vi "SRV_Strip Error if Matching Code.vi"(3 "error in (no error)":errorcluster, 4 "Strip Codes":i32[](array[numeric])) -> (10 "error out":errorcluster)   [LabVIEW 2014]
doc: "Strips the error if \"error in (code)\" matches one of the Strip Codes.\n\n\nAuthor: Mike Schultz - Logic PD"
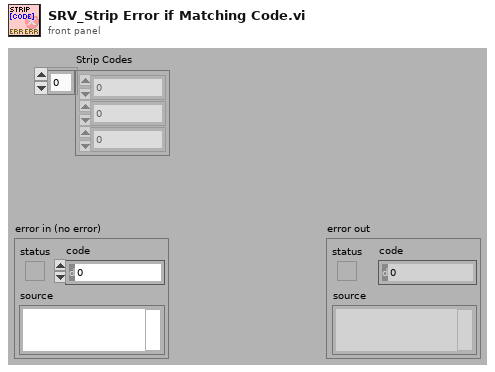
[diagram p1: front panel]
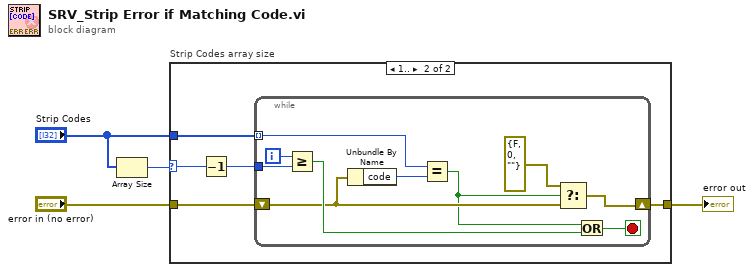
[diagram p0: block diagram]
diagram:
  n1 = Array Size(array="Strip Codes") -> (size(s)=w4:i32)
  n2 = case "Strip Codes array size" shown="1.." w4 {
    selector: w4 -> [_ w6]
    tunnel: "Strip Codes" -> [_ w10]
    tunnel: "error in (no error)" -> [w5 w9]
    tunnel: [w5 w8] -> w1
    frame ..0 {
    }
    frame 1.. {
      n3 = Decrement(x=w6) -> (x-1=w7:i32)
      n4 = while {
        tunnel: w7 -> [w17]
        shift-left: w9 -> [w14]
        shift-right: [w13] -> w8
        tunnel: w10 -> [w16] mode=indexing
        i -> [w18]
        stop <- w20 stop-if-true
        n5 = Greater Or Equal?(x=w18, y=w17) -> (x >= y?=w19:bool)
        n6 = Unbundle By Name(w14) -> ("code"=w15:i32)
        n7 = Equal?(x=w16, y=w15) -> (x = y?=w12:bool)
        n8 = Select(t=errorcluster {"status"=FALSE, "code"=0, "source"=""}, s=w12, f=w14) -> (s? t:f=w13:errorcluster)
        n9 = Or(x=w12, y=w19) -> (x .or. y?=w20:bool)
      }
    }
  }
  "error out" <- w1
